vi "Add Protection.vi"(8 "error in (no error)":errorcluster, 9 "Pad":bool, 10 "String in":string, 11 "CRC-32 in":refnum<class "CRC-32.lvclass">) -> (0 "error out":errorcluster, 2 "String out":string, 3 "CRC-32 out":refnum<class "CRC-32.lvclass">)   [LabVIEW 2013, in "Protections.lvlib" / "CRC-32.lvclass"]
uses:
  CRC-32.lvclass
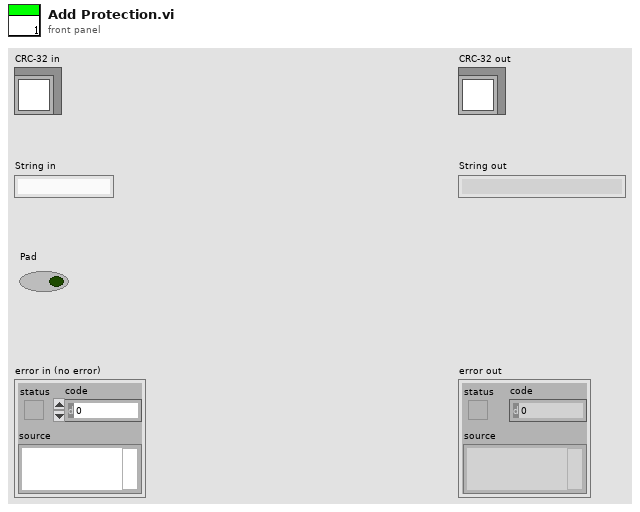
[diagram p1: front panel]
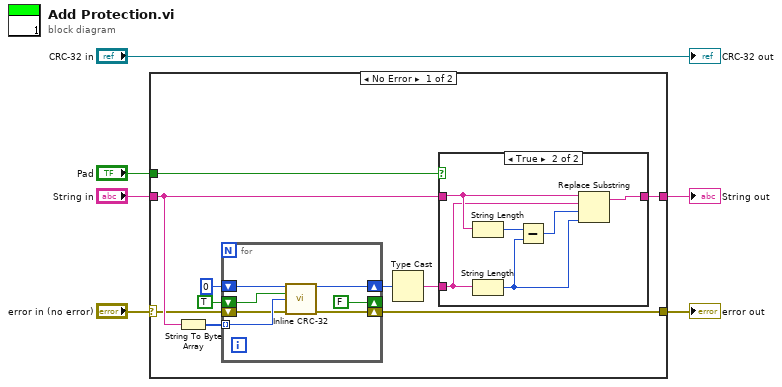
[diagram p0: block diagram]
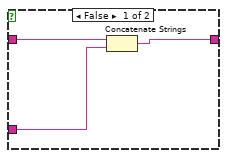
[diagram p2: hidden frame]
diagram:
  n1 = case shown="No Error" "error in (no error)" {
    selector: "error in (no error)" -> [w7 w34]
    tunnel: [w16 w33] -> w6
    tunnel: "String in" -> [w15 w33]
    tunnel: "Pad" -> [w14 _]
    tunnel: [w10 w34] -> w2
    frame No Error {
      n2 = String To Byte Array(string=w15) -> (unsigned byte array=w12:u8[])
      n3 = for {
        shift-right: [w22] -> w9
        shift-left: u32 0 ("CRC") -> [w23]
        tunnel: w12 -> [w21] mode=indexing
        shift-right: [w19] -> w10
        shift-left: w7 -> [w20]
        shift-right: [FALSE] -> _
        shift-left: TRUE -> [w18]
        n4 = call "Inline CRC-32.vi"("CRC In"=w23, "Reset"=w18, "Data"=w21, "error in (no error)"=w20) -> ("CRC"=w22:u32, "error out"=w19:errorcluster)  [unwired: 10 in]
      }
      n5 = Type Cast(x=w9) -> (*(type *) &x=w8:string)  [unwired: 1 in]
      n6 = case shown="True" w14 {
        tunnel: w8 -> [w26 w27]
        tunnel: w15 -> [w25 w31]
        tunnel: [w24 w32] -> w16
        frame False {
          n7 = Concatenate Strings(w25, w26) -> (w24:string)
        }
        frame True {
          n8 = String Length(string=w31) -> (length=w30:i32)
          n9 = String Length(string=w27) -> (length=w29:i32)
          n10 = Subtract(x=w30, y=w29) -> (x-y=w28:i32)
          n11 = Replace Substring(2:w29, 3:w28, 4:w27, 5:w31) -> (1:w32:string)  [unwired: 1 out]
        }
      }
    }
    frame Error {
    }
  }
  "error out" <- w2
  "String out" <- w6
  "CRC-32 out" <- "CRC-32 in"
